vi "Main.vi"() -> ()   [LabVIEW 2020]
uses:
  C:/Program Files/Newport/Piezo Motion Control/Newport AG-UC2-UC8 Applet/Samples/LabVIEW 2009/AgilisCmdLib.dll
  Program Files/Newport/Piezo Motion Control/Newport AG-UC2-UC8 Applet/Samples/LabVIEW 2009/AgilisCmdLib.dll
panel:
  in  "ChannelNumber":i32=2
  in  "Stop":bool
  out "Moving":bool
  out "axis":i32
  in  "Axis number":string(combo)
  in  "Center":bool
  in  "Calibrate":bool
  in  "previousPosition":dbl
  in  "newPosition":dbl caption="Offset (mm)" min=-10.0 max=10.0 format="%.6f"
  out "reference":refnum<k24>
  out "averageReverseStepSize":dbl caption="Average reverse step size (micron)"
  out "averageForwardStepSize":dbl caption="Average forward step size (micron)"
  out "travelRange":i32
  out "lastCalibration":string caption="Last calibration"
  in  "Step amplitude":i32=1 min=10 max=50 step=1
  in  "COM port":string(combo)
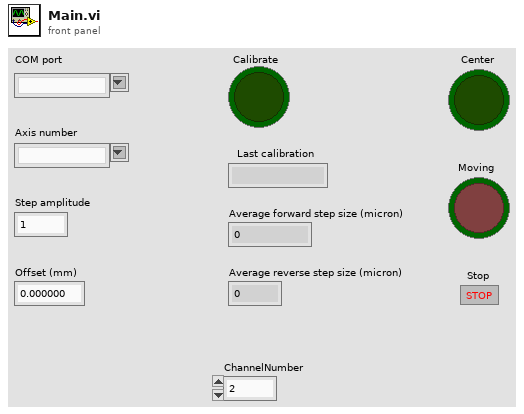
[diagram p1: front panel]
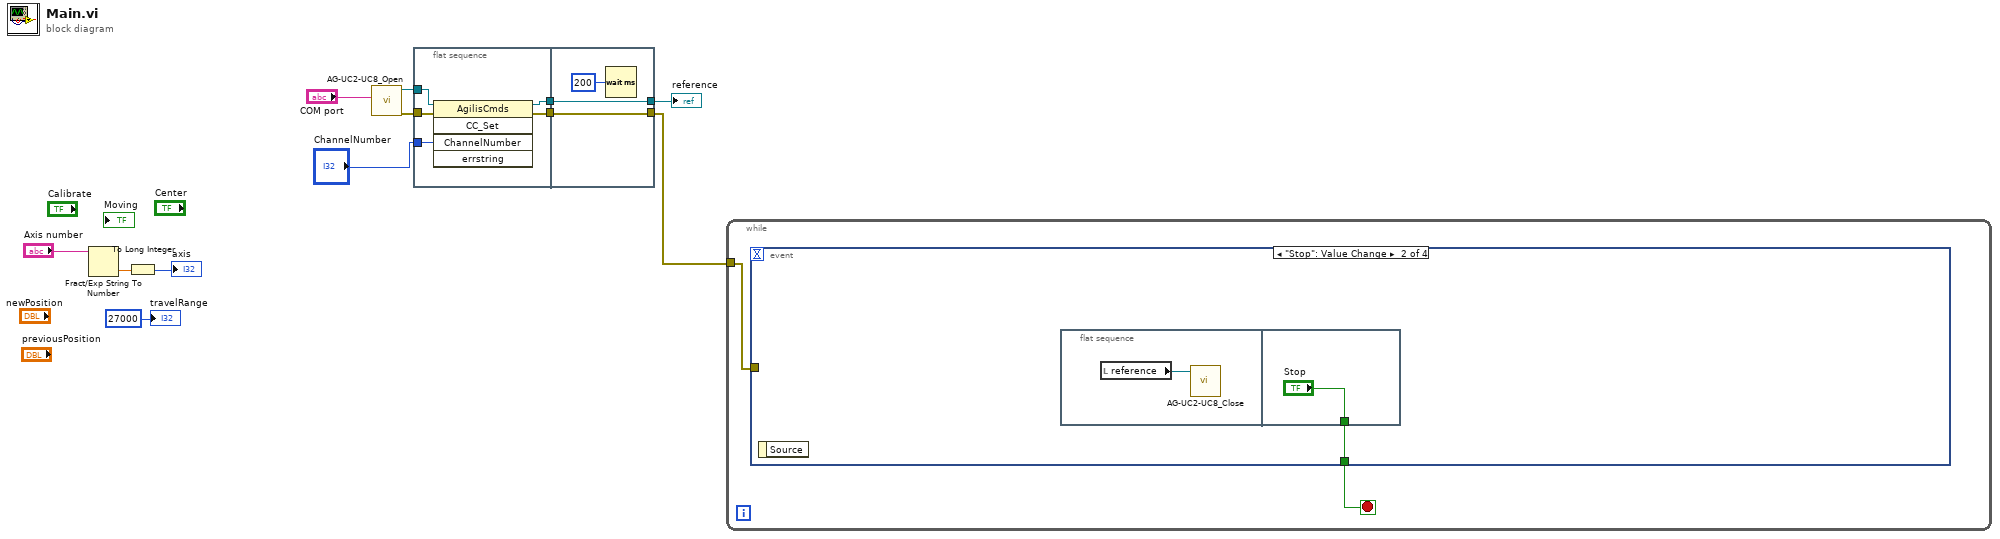
[diagram p0: block diagram]
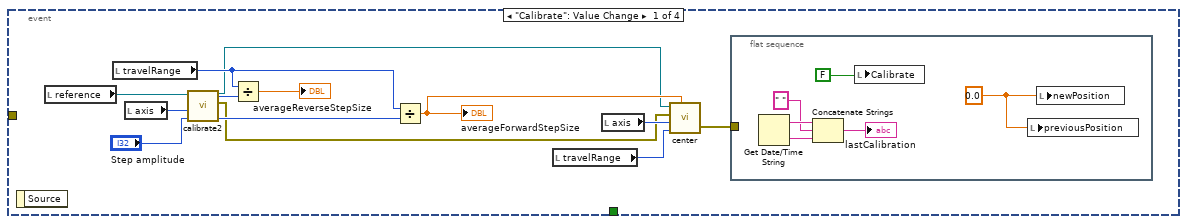
[diagram p2: hidden frame]
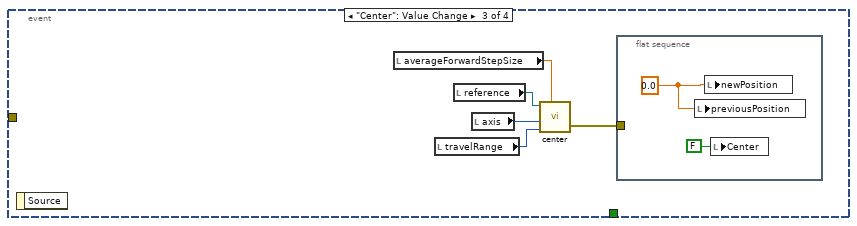
[diagram p3: hidden frame]
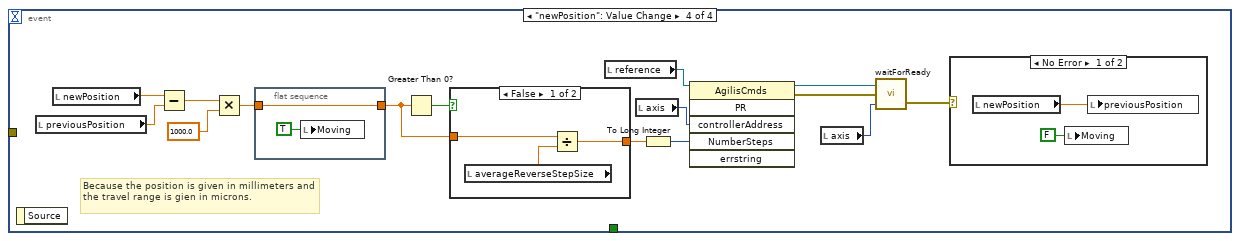
[diagram p4: hidden frame]
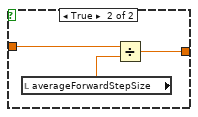
[diagram p6: hidden frame]
diagram:
  n1 = Fract/Exp String To Number(string="Axis number") -> (number=w11:dbl)  [unwired: 3 in, 1 out]
  n2 = To Long Integer(number=w11) -> (32bit integer=→"axis":i32)
  n3 = call "AG-UC2-UC8_Open.vi"("Instrument Key IN"="COM port") -> ("error out"=w5:errorcluster, "AG-UC2-UC8 Reference"=w2:refnum<k24>)  [unwired: 3 in, 2 out]
  n4 = flat-sequence {
    tunnel: [w17] -> w7
    tunnel: [w16] -> w6
    tunnel: w5 -> [w15]
    tunnel: w2 -> [w14]
    tunnel: "ChannelNumber" -> [w13]
    tunnel: w7 -> [w18]
    tunnel: w6 -> [w19]
    tunnel: [w19] -> w3
    tunnel: [w18] -> w1
    frame #0 {
      n5 = invoke class="AgilisCmds" method="CC_Set"(reference=w14, error in=w15, "ChannelNumber"=w13) -> (reference out=w17:refnum<k24>, error out=w16:errorcluster)  [unwired: 2 in, 3 out]
    }
    frame #1 {
      n6 = Wait (ms)(milliseconds to wait=u32 200) -> ()  [unwired: 1 out]
    }
  }
  n7 = while {
    tunnel: w3 -> [w22]
    stop <- w21 stop-if-true
    n8 = event shown="[1] \"Stop\": Value Change" {
      selector: _ -> [_ _ _ _]
      dyn-events: _ -> [_ _ _ _]
      timeout: _ -> [_ _ _ _]
      tunnel: w22 -> [_ _ _ _]
      tunnel: [_ w42 _ _] -> w21
      event "Calibrate": Value Change {
        n9 = event-data() -> ()  [unwired: 1 in, 1 out]
        n10 = local read "reference"() -> (w35:refnum<k24>)
        n11 = local read "travelRange"() -> (w31:i32)
        n12 = local read "axis"() -> (w34:i32)
        n13 = call "calibrate2.vi"("stepAmp"="Step amplitude", "axis"=w34, "referenceIn"=w35) -> ("nForwardSteps"=w30:i32, "nReverseSteps"=w32:i32, "errorOut"=w23:errorcluster, "referenceOut"=w24:refnum<k24>)  [unwired: 1 in]
        n14 = Divide(x=w31, y=w32) -> (x/y=→"averageReverseStepSize":dbl)
        n15 = Divide(x=w31, y=w30) -> (x/y=w25:dbl)
        "averageForwardStepSize" <- w25
        n16 = local read "travelRange"() -> (w27:i32)
        n17 = local read "axis"() -> (w28:i32)
        n18 = call "center.vi"("referenceIn"=w24, "errorIn"=w23, "axis"=w28, "travelRange"=w27, "averageForwardStepSize"=w25) -> ("errorOut"=w26:errorcluster)  [unwired: 1 out]
        n19 = flat-sequence {
          tunnel: w26 -> [_]
          frame #0 {
            w41 = 0.0 ("Position (mm)")
            n20 = Get Date/Time String() -> (date string=w40:string, time string=w39:string)  [unwired: 3 in]
            n21 = Concatenate Strings(w40, " " ("string"), w39) -> (→"lastCalibration":string)
            n22 = local write "Calibrate"(FALSE ("Calibrate")) -> ()
            n23 = local write "previousPosition"(w41) -> ()
            n24 = local write "newPosition"(w41) -> ()
          }
        }
      }
      event "Stop": Value Change {
        n25 = event-data() -> ()  [unwired: 1 in, 1 out]
        n26 = flat-sequence {
          tunnel: ["Stop"] -> w42
          frame #0 {
            n27 = local read "reference"() -> (w43:refnum<k24>)
            n28 = call "AG-UC2-UC8_Close.vi"("AG-UC2-UC8 Reference"=w43) -> ()  [unwired: 3 in, 2 out]
          }
          frame #1 {
          }
        }
      }
      event "Center": Value Change {
        n29 = event-data() -> ()  [unwired: 1 in, 1 out]
        n30 = local read "averageForwardStepSize"() -> (w48:dbl)
        n31 = local read "travelRange"() -> (w49:i32)
        n32 = local read "reference"() -> (w47:refnum<k24>)
        n33 = local read "axis"() -> (w46:i32)
        n34 = call "center.vi"("referenceIn"=w47, "axis"=w46, "travelRange"=w49, "averageForwardStepSize"=w48) -> ("errorOut"=w45:errorcluster)  [unwired: 1 in, 1 out]
        n35 = flat-sequence {
          tunnel: w45 -> [_]
          frame #0 {
            w51 = 0.0 ("Position (mm)")
            n36 = local write "previousPosition"(w51) -> ()
            n37 = local write "newPosition"(w51) -> ()
            n38 = local write "Center"(FALSE ("Center")) -> ()
          }
        }
      }
      event "newPosition": Value Change {
        # "Because the position is given in millimeters and the travel range is gien in microns."
        n39 = event-data() -> ()  [unwired: 1 in, 1 out]
        n40 = local read "previousPosition"() -> (w65:dbl)
        n41 = local read "newPosition"() -> (w66:dbl)
        n42 = Subtract(x=w66, y=w65) -> (x-y=w57:dbl)
        n43 = Multiply(x=w57, y=1000.0) -> (x*y=w55:dbl)
        n44 = flat-sequence {
          tunnel: w55 -> [w67]
          tunnel: [w67] -> w54
          frame #0 {
            n45 = local write "Moving"(TRUE ("Moving")) -> ()
          }
        }
        n46 = Greater Than 0?(x=w54) -> (x > 0?=w64:bool)
        n47 = case shown="False" w64 {
          tunnel: w54 -> [w73 w76]
          tunnel: [w71 w74] -> w53
          frame False {
            n48 = local read "averageReverseStepSize"() -> (w72:dbl)
            n49 = Divide(x=w73, y=w72) -> (x/y=w71:dbl)
          }
          frame True {
            n50 = local read "averageForwardStepSize"() -> (w75:dbl)
            n51 = Divide(x=w76, y=w75) -> (x/y=w74:dbl)
          }
        }
        n52 = local read "reference"() -> (w63:refnum<k24>)
        n53 = local read "axis"() -> (w62:i32)
        n54 = To Long Integer(number=w53) -> (32bit integer=w52:i32)
        n55 = invoke class="AgilisCmds" method="PR"(reference=w63, "controllerAddress"=w62, "NumberSteps"=w52) -> (reference out=w59:refnum<k24>, error out=w61:errorcluster)  [unwired: 3 in, 4 out]
        n56 = local read "axis"() -> (w60:i32)
        n57 = call "waitForReady.vi"("axis"=w60, "errorIn"=w61, "referenceIn"=w59) -> ("errorOut"=w58:errorcluster)  [unwired: 1 out]
        n58 = case shown="No Error" w58 {
          frame No Error {
            n59 = local read "newPosition"() -> (w70:dbl)
            n60 = local write "Moving"(FALSE ("Moving")) -> ()
            n61 = local write "previousPosition"(w70) -> ()
          }
          frame Error {
          }
        }
      }
    }
  }
  "travelRange" <- 27000 ("travelRange")
  "reference" <- w1
